vi "TangoPositions2MultiList.vi"(8 "error in (no error)":errorcluster, 11 "Saved Positions":T1(array[cluster])) -> (0 "error out":errorcluster, 3 "Array":string[][](array[string]))   [LabVIEW 2018, in "TangoOWN.lvlib"]
uses:
  TangoOWN.lvlib
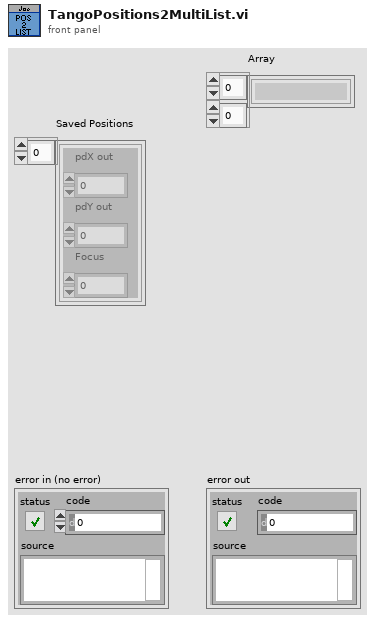
[diagram p1: front panel]
types:
  T1 = cluster{"pdX out":dbl, "pdY out":dbl, "Focus":dbl}[]
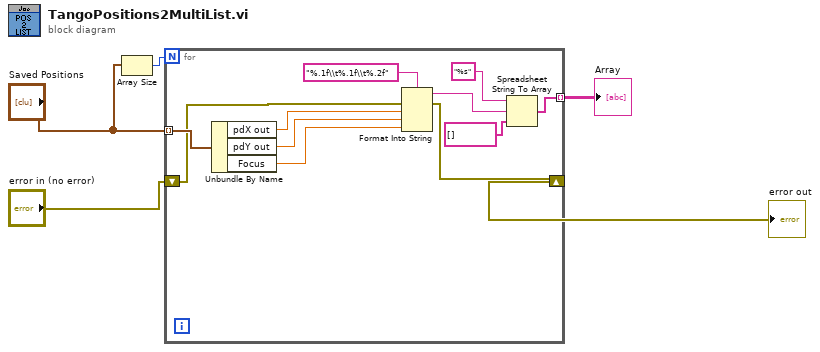
[diagram p0: block diagram]
diagram:
  n1 = Array Size(array="Saved Positions") -> (size(s)=w2:i32)
  n2 = for {
    N: w2 -> [_]
    tunnel: "Saved Positions" -> [w16] mode=indexing
    tunnel: [w7] -> w5 mode=indexing
    shift-right: [w10] -> w4
    shift-left: "error in (no error)" -> [w12]
    n3 = Unbundle By Name(w16) -> ("pdX out"=w15:dbl, "pdY out"=w14:dbl, "Focus"=w13:dbl)
    n4 = Format Into String(format string="%.1f\\t%.1f\\t%.2f", error in=w12, w15, w14, w13) -> (resulting string=w9:string, error out=w10:errorcluster)  [unwired: 1 in]
    n5 = Spreadsheet String To Array(format string="%s", spreadsheet string=w9, array type (2D Dbl)=string[] []) -> (array=w7:string[])  [unwired: 1 in]
  }
  "Array" <- w5
  "error out" <- w4
